vi "DAE Spring Pendulum Simulation_Draw Spring.vi"(6 "width":dbl=10.0, 8 "color(blue)":u32(colorbox)=590024, 9 "End point":cluster{"x":i16, "y":i16}={"x"=200, "y"=200}, 10 "Start point":cluster{"x":i16, "y":i16}={"x"=200, "y"=200}, 11 "picture in":picture) -> (3 "picture out":picture)   [LabVIEW 2023]
doc: "DAE Spring Pendulum Simulation Draw Spring"
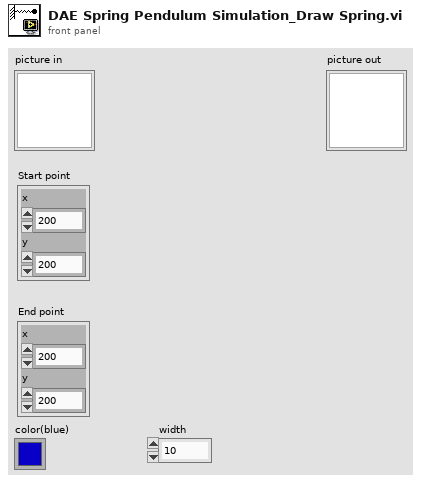
[diagram p1: front panel]
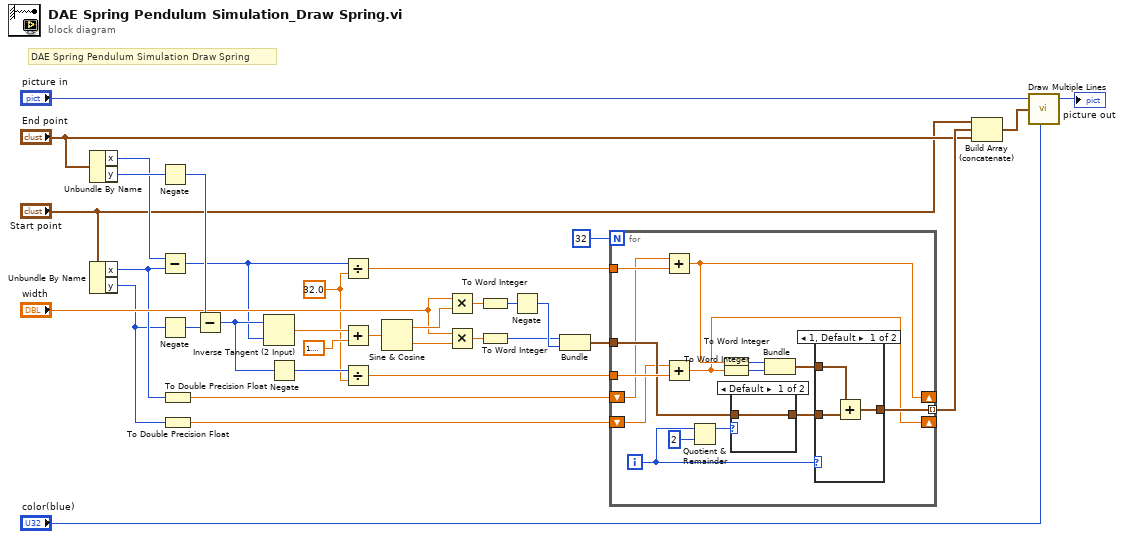
[diagram p0: block diagram]
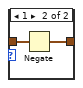
[diagram p3: hidden frame]
diagram:
  w1 = 32.0 ("y")
  # "DAE Spring Pendulum Simulation Draw Spring"
  n1 = Unbundle By Name("End point") -> ("x"=w33:i16, "y"=w34:i16)
  n2 = Unbundle By Name("Start point") -> ("x"=w9:i16, "y"=w7:i16)
  n3 = Negate(x=w34) -> (-x=w32:i16)
  n4 = Subtract(x=w33, y=w9) -> (x-y=w4:i16)
  n5 = Negate(x=w7) -> (-x=w23:i16)
  n6 = To Double Precision Float(number=w9) -> (double precision float=w8:dbl)
  n7 = To Double Precision Float(number=w7) -> (double precision float=w6:dbl)
  n8 = Subtract(x=w32, y=w23) -> (x-y=w13:i16)
  n9 = Inverse Tangent (2 Input)(1:w4, 2:w13) -> (0:w27:dbl)
  n10 = Negate(x=w13) -> (-x=w2:i16)
  n11 = Divide(x=w4, y=w1) -> (x/y=w22:dbl)
  n12 = Add(x=w27, y=1.5707963267948966) -> (x+y=w25:dbl)
  n13 = Divide(x=w2, y=w1) -> (x/y=w24:dbl)
  n14 = Sine & Cosine(0:w25) -> (1:w31:dbl, 2:w30:dbl)
  n15 = Multiply(x="width", y=w31) -> (x*y=w29:dbl)
  n16 = Multiply(x="width", y=w30) -> (x*y=w28:dbl)
  n17 = To Word Integer(number=w29) -> (16bit integer=w19:i16)
  n18 = To Word Integer(number=w28) -> (16bit integer=w17:i16)
  n19 = Negate(x=w19) -> (-x=w18:i16)
  n20 = Bundle(w17, w18) -> (w21:cluster{i16, i16})  [unwired: 1 out]
  n21 = for {
    N: 32 -> [_]
    tunnel: w24 -> [w49]
    tunnel: w22 -> [w48]
    tunnel: w21 -> [w40]
    tunnel: [w46] -> w16 mode=indexing
    shift-right: [w37] -> _
    shift-left: w8 -> [w38]
    shift-right: [w35] -> _
    shift-left: w6 -> [w36]
    i -> [w39]
    n22 = Add(x=w38, y=w48) -> (x+y=w37:dbl)
    n23 = Add(x=w36, y=w49) -> (x+y=w35:dbl)
    n24 = Quotient & Remainder(x=w39, y=2) -> (x-y*floor(x/y)=w42:i32)  [unwired: 1 out]
    n25 = To Word Integer(number=w37) -> (16bit integer=w45:i16)
    n26 = To Word Integer(number=w35) -> (16bit integer=w44:i16)
    n27 = case shown="Default" w42 {
      tunnel: [w54 w55] -> w41
      tunnel: w40 -> [w54 w56]
      frame Default {
      }
      frame 1 {
        n28 = Negate(x=w56) -> (-x=w55:cluster{i16, i16})
      }
    }
    n29 = Bundle(w45, w44) -> (w47:cluster{i16, i16})  [unwired: 1 out]
    n30 = case shown="1, Default" w39 {
      tunnel: w47 -> [w52 w53]
      tunnel: [w51 w53] -> w46
      tunnel: w41 -> [w50 _]
      frame 1, Default {
        n31 = Add(x=w52, y=w50) -> (x+y=w51:cluster{i16, i16})
      }
      frame 0, 30, 31 {
      }
    }
  }
  n32 = Build Array (concatenate)("Start point", w16, "End point") -> (w15:cluster{"x":i16, "y":i16}[])
  n33 = call <vilib>:"Draw Multiple Lines.vi"("picture"="picture in", "line endpoints"=w15, "color(black)"="color(blue)") -> ("new picture"=→"picture out":picture)  [unwired: 2 in, 4 out]
